vi "GetControlPath.vi"(11 "Error control type":T1) -> (2 "Exists?":bool, 3 "Path":path)   [LabVIEW 2017, in "ErrorStructureDrawer.lvlib"]
doc: "Returns the path to the error control for the specified type.\n\nIf an unhandled type is selected (e.g. System), or if no control is found for the specified type, then the path to the Modern error control is returned."
uses:
  Controls/ErrorControlType.ctl
  ErrorStructureDrawer.lvlib
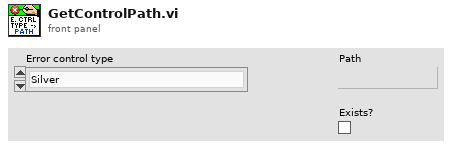
[diagram p1: front panel]
types:
  T1 = typedef "ErrorStructureDrawer.lvlib/ErrorControlType.ctl" = enum16{"Silver", "Modern", "Classic", "LabVIEW default", "NXG"}
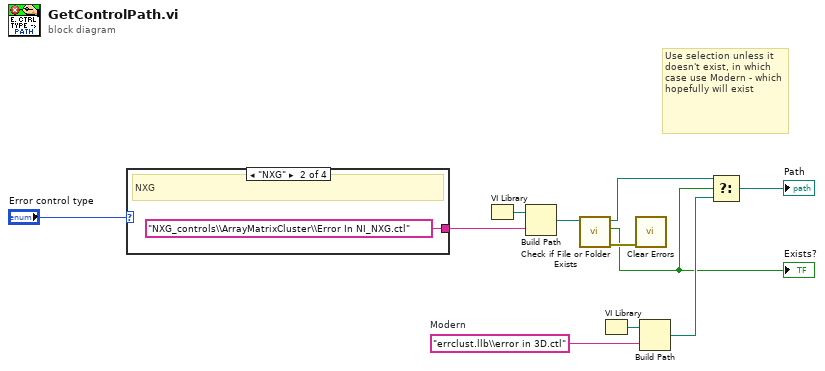
[diagram p0: block diagram]
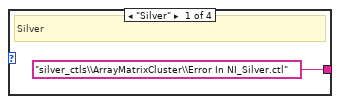
[diagram p2: hidden frame]
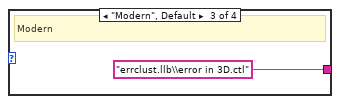
[diagram p3: hidden frame]
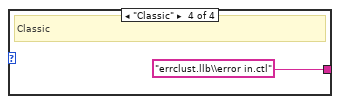
[diagram p4: hidden frame]
diagram:
  w5 = "errclust.llb\\error in 3D.ctl"  # Modern
  # "Use selection unless it doesn't exist, in which case use Modern - which hopefully will exist"
  n1 = case shown="\"NXG\"" "Error control type" {
    tunnel: ["silver_ctls\\ArrayMatrixCluster\\Error In NI_Silver.ctl" ("name or relative path") "NXG_controls\\ArrayMatrixCluster\\Error In NI_NXG.ctl" ("name or relative path") "errclust.llb\\error in 3D.ctl" ("name or relative path") "errclust.llb\\error in.ctl" ("name or relative path")] -> w8
    frame "Silver" {
      # "Silver"
    }
    frame "NXG" {
      # "NXG"
    }
    frame "Modern", Default {
      # "Modern"
    }
    frame "Classic" {
      # "Classic"
    }
  }
  n2 = VI Library() -> (path=w7:path)
  n3 = Build Path(base path=w7, name or relative path=w8) -> (appended path=w10:path)
  n4 = call <vilib>:"Check if File or Folder Exists.vi"("path"=w10) -> ("error out"=w11:errorcluster, "file or folder exists?"=w1:bool, "dup path"=w2:path)  [unwired: 8 in]
  "Exists?" <- w1
  n5 = VI Library() -> (path=w6:path)
  n6 = call <vilib>:"Clear Errors.vi"("error in (no error)"=w11) -> ()  [unwired: 5 in, 2 out]
  n7 = Build Path(base path=w6, name or relative path=w5) -> (appended path=w4:path)
  n8 = Select(t=w2, s=w1, f=w4) -> (s? t:f=→"Path":path)
